vi "GetCameraData.vi"(8 "error in (no error)":errorcluster, 9 "unit":string, 10 "Current Camera":string, 11 "Map":T1) -> (0 "error out":errorcluster, 3 "DataSet":T2)   [LabVIEW 2017, in "IrTestPanel.lvlib"]
uses:
  <vilib>/addons/InsightCM/Devices/Shared/Ir/IrTestPanel/IrTestPanel.lvlib
  <vilib>/addons/InsightCM/MessageBus/Base/controls/DataSetByteData.ctl
  <vilib>/addons/InsightCM/MessageBus/Base/controls/KeyValuePair.ctl
  <vilib>/addons/PointValueMap/controls/PointMap.ctl
  <vilib>/addons/InsightCM/Utilities/PropertyHelpers/PropertyHelpers.lvlib
  <vilib>/addons/PointValueMap/PointValueMap.lvlib
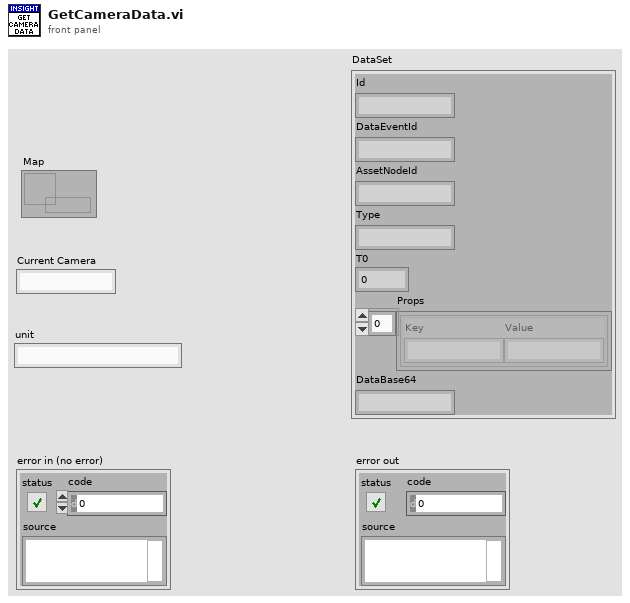
[diagram p1: front panel]
types:
  T1 = typedef "PointValueMap.lvlib/PointMap.ctl" = refnum<data-value>
  T2 = typedef "DataSetByteData.ctl" = cluster{"Id":string, "DataEventId":string, "AssetNodeId":string, "Type":string, "T0":i64, "Props":T3[], "DataBase64":string}
  T3 = typedef "KeyValuePair.ctl" = cluster{"Key":string, "Value":string}
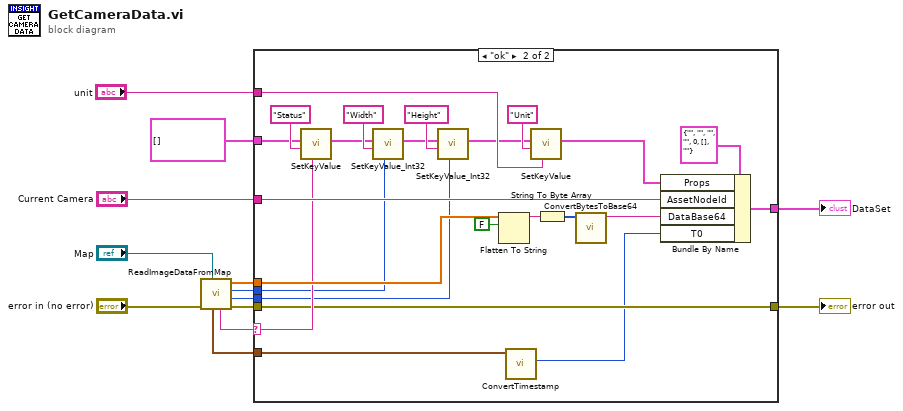
[diagram p0: block diagram]
diagram:
  n1 = call <vilib>:"ReadImageDataFromMap.vi"("map"="Map", "error in (no error)"="error in (no error)") -> ("error out"=w6:errorcluster, "image height"=w2:i32, "image width"=w3:i32, "image data"=w8:sgl[], "image status"=w9:string, "image timestamp"=w7:timestamp)  [unwired: 3 in, 1 out]
  n2 = case shown="\"ok\"" w9 {
    selector: w9 -> [_ w25]
    tunnel: [w14 w23] -> w12
    tunnel: "Current Camera" -> [_ w38]
    tunnel: [_ w36] -> w11
    tunnel: "unit" -> [_ w32]
    tunnel: w8 -> [_ w26]
    tunnel: w7 -> [_ w24]
    tunnel: w6 -> [w14 w23]
    tunnel: w3 -> [_ w16]
    tunnel: w2 -> [_ w15]
    tunnel: T3[] [] ("key value pairs") -> [_ w21]
    frame Default {
    }
    frame "ok" {
      n3 = call <vilib>:"SetKeyValue.vi"("value"=w25, "key"="Status", "key value pairs"=w21) -> ("key value pairs out"=w20:T3[])  [unwired: 8 in]
      n4 = call <vilib>:"SetKeyValue_Int32.vi"("value"=w16, "key"="Width", "key value pairs"=w20) -> ("key value pairs out"=w19:T3[])  [unwired: 8 in]
      n5 = call <vilib>:"SetKeyValue_Int32.vi"("value"=w15, "key"="Height", "key value pairs"=w19) -> ("key value pairs out"=w18:T3[])  [unwired: 8 in]
      n6 = Flatten To String(anything=w26, prepend array or string size? (T)=FALSE) -> (data string=w29:string)  [unwired: 2 in, 2 out]
      n7 = call <vilib>:"ConvertTimestamp.vi"("Time Stamp"=w24) -> ("Timestamp out"=w22:i64)  [unwired: 10 in]
      n8 = call <vilib>:"SetKeyValue.vi"("value"=w32, "key"="Unit", "key value pairs"=w18) -> ("key value pairs out"=w17:T3[])  [unwired: 8 in]
      n9 = String To Byte Array(string=w29) -> (unsigned byte array=w31:u8[])
      n10 = call <vilib>:"ConvertBytesToBase64.vi"("U8 array"=w31) -> ("base64 encoded"=w27:string)  [unwired: 10 in]
      n11 = Bundle By Name(cluster=T2 {"Id"="", "DataEventId"="", "AssetNodeId"="", "Type"="", "T0"=0, "Props"=[], "DataBase64"=""} ("DataSet"), "Props"=w17, "AssetNodeId"=w38, "DataBase64"=w27, "T0"=w22) -> (w36:T2)
    }
  }
  "error out" <- w12
  "DataSet" <- w11
